vi "Noyito10ChannelADC_ConfigSerialPort&Connect.vi"(8 "error in (no error)":errorcluster) -> (0 "error out":errorcluster, 3 "Noyito 10Chan ADC Mod":refnum<visa-resource-name>)   [LabVIEW 2020]
uses:
  <vilib>/Instr/_visa.llb/VISA Configure Serial Port (Instr).vi
panel:
  out "userMessage":string
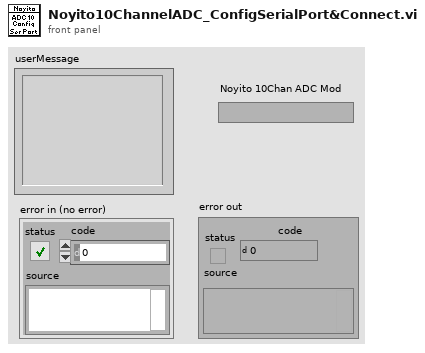
[diagram p1: front panel]
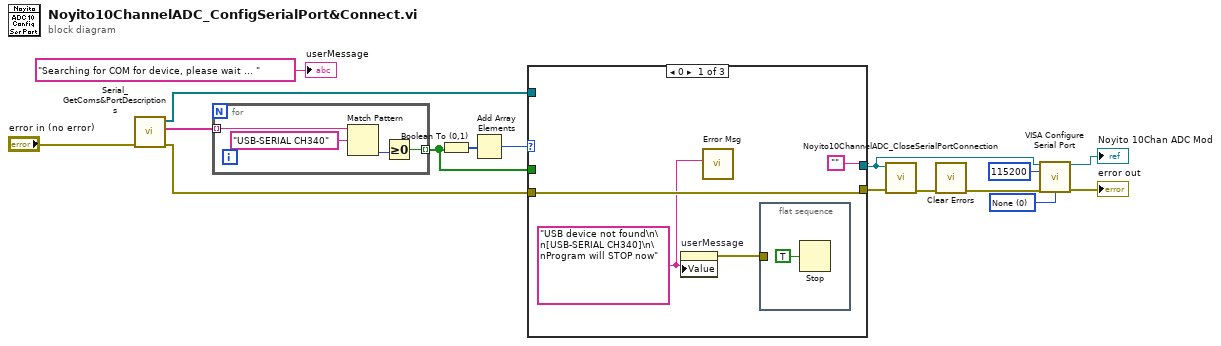
[diagram p0: block diagram]
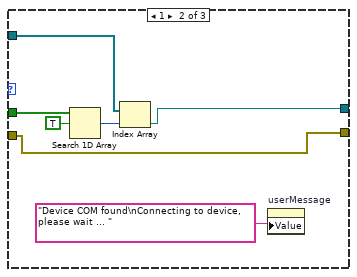
[diagram p2: hidden frame]
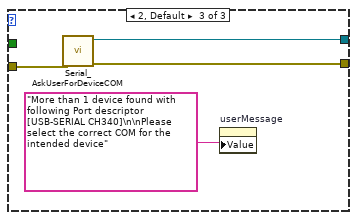
[diagram p3: hidden frame]
diagram:
  w8 = u16 0 items=["None", "XON/XOFF", "RTS/CTS", "XON/XOFF & RTS/CTS", "DTR/DSR", "XON/XOFF & DTR/DSR"] ("flow control (0:none)")
  n1 = call "Serial_GetComs&PortDescriptions.vi"("error in (no error)"="error in (no error)") -> ("error out"=w12:errorcluster, "WinsDescriptions"=w16:string[], "COMs"=w10:refnum<visa-resource-name>[])  [unwired: 8 in]
  n2 = for {
    tunnel: w16 -> [w20] mode=indexing
    tunnel: [w17] -> w11 mode=indexing
    n3 = Match Pattern(string=w20, regular expression="USB-SERIAL CH340") -> (offset past match=w18:i32)  [unwired: 1 in, 3 out]
    n4 = Greater Or Equal To 0?(x=w18) -> (x >= 0?=w17:bool)
  }
  n5 = Boolean To (0,1)(Boolean=w11) -> (0, 1=w15:i16[])
  n6 = Add Array Elements(numeric array=w15) -> (sum=w14:i16)
  n7 = case shown="0" w14 {
    tunnel: w12 -> [w23 w26 w35]
    tunnel: [w23 w26 w34] -> w4
    tunnel: ["" w27 w33] -> w1
    tunnel: w11 -> [_ w31 _]
    tunnel: w10 -> [_ w28 _]
    frame 0 {
      w21 = "USB device not found\n\n[USB-SERIAL CH340]\n\nProgram will STOP now" ("regular expression")
      n8 = property on="userMessage" class="Str"("Value"=w21) -> (error out=w24:errorcluster)  [unwired: 2 in, 1 out]
      n9 = call "Error Msg"("Message"=w21) -> ()  [unwired: 9 in, 2 out]
      n10 = flat-sequence {
        tunnel: w24 -> [_]
        frame #0 {
          n11 = Stop(stop? (T)=TRUE) -> ()
        }
      }
    }
    frame 1 {
      n12 = Search 1D Array(1D array=w31, element=TRUE) -> (index of element=w29:i32)  [unwired: 1 in]
      n13 = Index Array(array=w28, index=w29) -> (element=w27:refnum<visa-resource-name>)
      n14 = property on="userMessage" class="Str"("Value"="Device COM found\nConnecting to device, please wait ... " ("regular expression")) -> ()  [unwired: 2 in, 2 out]
    }
    frame 2, Default {
      n15 = call "Serial_AskUserForDeviceCOM.vi"("error in (no error)"=w35) -> ("error out"=w34:errorcluster, "Com-Out"=w33:refnum<visa-resource-name>)  [unwired: 9 in]
      n16 = property on="userMessage" class="Str"("Value"="More than 1 device found with following Port descriptor [USB-SERIAL CH340]\n\nPlease select the correct COM for the intended device" ("regular expression")) -> ()  [unwired: 2 in, 2 out]
    }
  }
  n17 = call "Noyito10ChannelADC_CloseSerialPortConnection.vi"("error in (no error)"=w4, "Noyito 10Chan ADC Mod"=w1) -> ("error out"=w3:errorcluster)  [unwired: 8 in, 1 out]
  n18 = call <vilib>:"Clear Errors.vi"("error in (no error)"=w3) -> ("error out"=w2:errorcluster)  [unwired: 5 in, 1 out]
  n19 = call-poly "VISA Configure Serial Port"("VISA resource name"=w1, "baud rate (9600)"=u32 115200, "error in (no error)"=w2, "flow control (0:none)"=w8) -> ("VISA resource name out"=→"Noyito 10Chan ADC Mod":refnum<visa-resource-name>, "error out"=→"error out":errorcluster)  [unwired: 10 in]
  "userMessage" <- "Searching for COM for device, please wait ... " ("regular expression")
